vi "Test - Draw Filled Triangle 1D.vi"() -> ()   [LabVIEW 2020, in "Raster.lvlib"]
uses:
  Raster.lvlib
  3D/Triangle.ctl
  3D/Vertex.ctl
  3D/Vector 3D.ctl
  UV.ctl
  3D/Material.ctl
  Texture.ctl
  Rectangle Dimensions.ctl
  5ea285c7-be76-47ab-bb95-511c6a9aac96.vi
  d84cddbd-8e40-43c7-a758-6e8d8fd6f2c6.vi
  <vilib>/Utility/High Resolution Relative Seconds.vi
  3D/Calc Index.vi
  Calc Pixel Row Stats.vi
  Check Is Middle Reached.vi
  Sort Points.vi
  Calculate Pixel Reciprocals.vi
  Calc Pixel Starting Conditions.vi
  Round SGL.vi
  Utility/Convert Pixels To Picture.vi/d601d993-a776-4dc8-89c7-357d8398c88c.vi
  Utility/Convert Pixels To Picture.vi/7816d0d6-8e4d-41a2-85ac-ed82f1435763.vi
  3D/Round Vertex.vi
  Calculate Line Reciprocal.vi
  Check Is Triangle Flat Bottomed.vi
  Global 1.vi
  <vilib>/picture/picture.llb/Draw Unflattened Pixmap.vi
  <vilib>/picture/picture.llb/Draw True-Color Pixmap.vi
  Utility/Utility.lvlib
  3D/3D.lvlib
panel:
  in  "Triangle":T1={"Vertex 1"={"Position"={"x"=75.0, "y"=25.0, "z"=0.0}, "UV"={"u"=0.0, "v"=0.0}, "Colour"=12517256}, "Vertex 2"={"Position"={"x"=500.0, "y"=450.0, "z"=0.0}, "UV"={"u"=0.0, "v"=0.0}, "Colour"=12517256}, "Vertex 3"={"Position"={"x"=50.0, "y"=200.0, "z"=0.0}, "UV"={"u"=0.0, "v"=0.0}, "Colour"=12517256}, "Alpha"=0.0, "Alpha Blending Enabled"=FALSE, "Colour"=10092492, "Material"={"Diffuse Colour"=0, "Texture"={"Pixels"=refnum, "Size"={"Width"=0, "Height"=0}}}} {"Vertex 3"."UV"."v" min=0 max=1 step=0.1; "Vertex 3"."UV"."u" min=0 max=1 step=0.1; "Vertex 2"."UV"."v" min=0 max=1 step=0.1; "Vertex 2"."UV"."u" min=0 max=1 step=0.1; "Vertex 1"."UV"."v" min=0 max=1 step=0.1; "Vertex 1"."UV"."u" min=0 max=1 step=0.1}
  out "Time [s]":dbl format="%.3p"
  out "new picture":picture
  # "(0,0)"
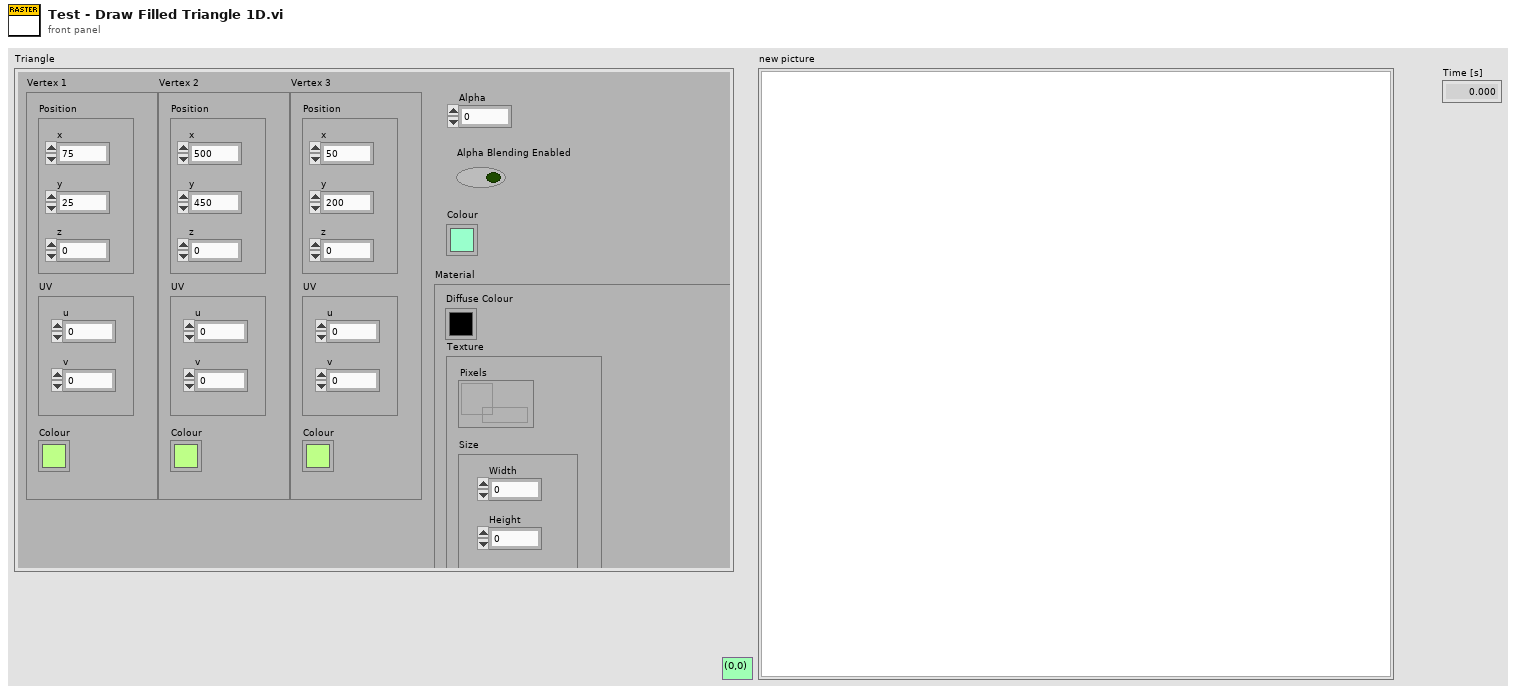
[diagram p1: front panel]
types:
  T1 = typedef "3D.lvlib/Triangle.ctl" = cluster{"Vertex 1":T2, "Vertex 2":T2, "Vertex 3":T2, "Alpha":dbl, "Alpha Blending Enabled":bool, "Colour":u32, "Material":T5}
  T2 = typedef "3D.lvlib/Vertex.ctl" = cluster{"Position":T3, "UV":T4, "Colour":u32}
  T3 = typedef "3D.lvlib/Vector 3D.ctl" = cluster{"x":sgl, "y":sgl, "z":sgl}
  T4 = typedef "Raster.lvlib/UV.ctl" = cluster{"u":sgl, "v":sgl}
  T5 = typedef "3D.lvlib/Material.ctl" = cluster{"Diffuse Colour":u32, "Texture":T6}
  T6 = typedef "Raster.lvlib/Texture.ctl" = cluster{"Pixels":refnum<data-value>, "Size":T7}
  T7 = typedef "Raster.lvlib/Rectangle Dimensions.ctl" = cluster{"Width":u32, "Height":u32}
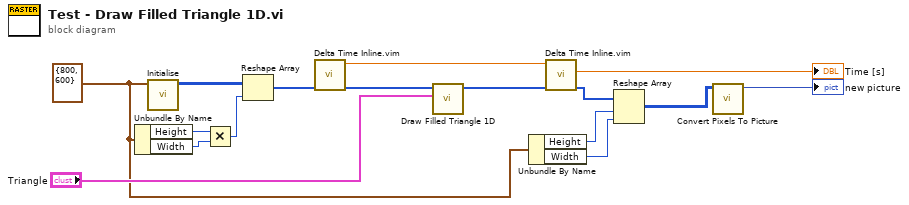
[diagram p0: block diagram]
diagram:
  w4 = T7 {"Width"=800, "Height"=600} ("Screen Dimensions")
  n1 = Unbundle By Name(w4) -> ("Height"=w8:u32, "Width"=w7:u32)
  n2 = call "Initialise.vi"("Screen Dimensions"=w4) -> ("Pixel Data out"=w10:u32[][])  [unwired: 10 in]
  n3 = Multiply(x=w8, y=w7) -> (x*y=w6:u32)
  n4 = Reshape Array(w10, w6) -> (w9:u32[])
  n5 = call "Delta Time Inline.vim"("value in"=w9) -> ("value out"=w15:u32[], "Relative Seconds out [s]"=w12:dbl)  [unwired: 8 in, 1 out]
  n6 = call "Draw Filled Triangle 1D.vi"("Triangle"="Triangle", "Pixel Data in"=w15) -> ("Pixel Data out"=w14:u32[])  [unwired: 9 in]
  n7 = Unbundle By Name(w4) -> ("Height"=w3:u32, "Width"=w2:u32)
  n8 = call "Delta Time Inline.vim"("value in"=w14, "Relative Seconds in [s]"=w12) -> ("value out"=w5:u32[], "Delta Time [s]"=→"Time [s]":dbl)  [unwired: 7 in, 1 out]
  n9 = Reshape Array(w5, w3, w2) -> (w1:u32[][])
  n10 = call "Convert Pixels To Picture.vi"("Pixel Data in"=w1) -> ("2D Picture"=→"new picture":picture)  [unwired: 9 in, 1 out]
